vi "dfd_Multirate Filter Param Estimation.vi"(5 "method":u16(ring)=2 items=["Kaiser Window", "Dolph-Chebyshev Window", "Equi-Ripple", "Positive Equi-Ripple"], 7 "multirate factor":i32=4, 8 "error in (no error)":errorcluster, 9 "option":enum16{"Normal", "Nyquist", "Alias free"}(ring), 10 "roll off":dbl format="%.2f", 11 "order":i32) -> (0 "error out":errorcluster, 1 "window param":cluster{"low cutoff freq: fl":dbl, "param":dbl} {"param" format="%.2f"}, 2 "band parameters":T1[](array[typedef]), 3 "new order":i32)   [LabVIEW 2017, in "NI_DigFilter_Process.lvlib"]
uses:
  <vilib>/addons/Digital Filter Design/NI_DigFilter_Process.lvlib
  <vilib>/addons/Digital Filter Design/_Objects.llb/DFD Adv Band Spec.ctl
  <vilib>/addons/Digital Filter Design/NI_DigFilterLicensed.lvlib
panel:
  in  "band 2":T1
  # "freq"
  # "amplitude"
  # "weight"
  # "freq"
  # "amplitude"
  # "weight"
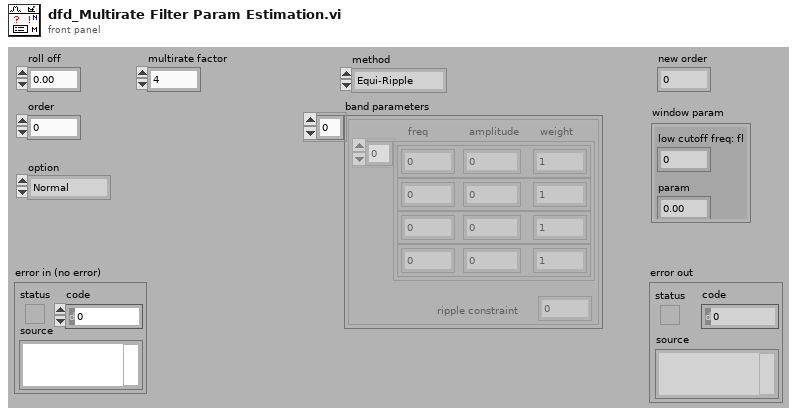
[diagram p1: front panel]
types:
  T1 = typedef "NI_DigFilterLicensed.lvlib/DFD Adv Band Spec.ctl" = cluster{"band specification":cluster{"freq":dbl, "amplitude":dbl, "weight":dbl}[], "ripple constraint":dbl}
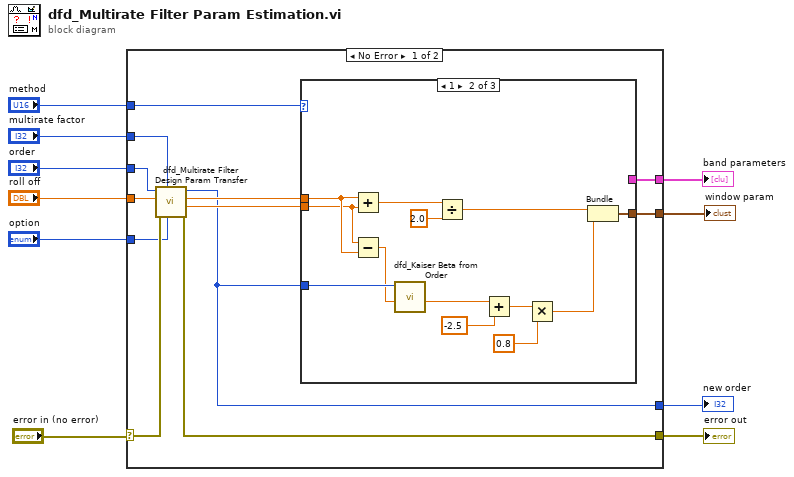
[diagram p0: block diagram]
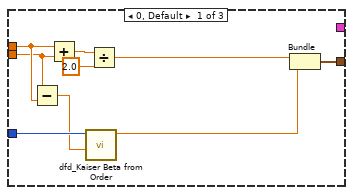
[diagram p2: hidden frame]
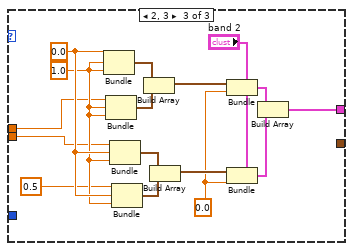
[diagram p3: hidden frame]
diagram:
  n1 = case shown="No Error" "error in (no error)" {
    selector: "error in (no error)" -> [w13 w61]
    tunnel: "roll off" -> [w18 _]
    tunnel: [w12 w61] -> w9
    tunnel: "method" -> [w22 _]
    tunnel: [w21 _] -> w7
    tunnel: "multirate factor" -> [w19 _]
    tunnel: "order" -> [w15 _]
    tunnel: [w20 _] -> w1
    tunnel: [w14 _] -> w3
    tunnel: "option" -> [w11 _]
    frame No Error {
      n2 = call <vilib>:"dfd_Multirate Filter Design Param Transfer.vi"("option"=w11, "multirate factor"=w19, "error in (no error)"=w13, "roll off"=w18, "order"=w15) -> ("error out"=w12:errorcluster, "fstop"=w17:dbl, "fpass"=w16:dbl, "new order"=w14:i32)  [unwired: 2 in, 1 out]
      n3 = case shown="1" w22 {
        tunnel: [_ _ w47] -> w21
        tunnel: w16 -> [w27 w40 w49]
        tunnel: w17 -> [w26 w39 w48]
        tunnel: w14 -> [w31 w44 _]
        tunnel: [w24 w37 _] -> w20
        frame 0, Default {
          n4 = Subtract(x=w26, y=w27) -> (x-y=w28:dbl)
          n5 = Add(x=w27, y=w26) -> (x+y=w29:dbl)
          n6 = call <vilib>:"dfd_Kaiser Beta from Order.vi"("delta f [Hz]"=w28, "order"=w31) -> ("beta"=w23:dbl)  [unwired: 9 out]
          n7 = Divide(x=w29, y=2.0) -> (x/y=w25:dbl)
          n8 = Bundle(w25, "beta"=w23) -> (w24:cluster{dbl, "beta":dbl})  [unwired: 1 out]
        }
        frame 1 {
          n9 = Add(x=w40, y=w39) -> (x+y=w42:dbl)
          n10 = Subtract(x=w39, y=w40) -> (x-y=w41:dbl)
          n11 = call <vilib>:"dfd_Kaiser Beta from Order.vi"("delta f [Hz]"=w41, "order"=w44) -> ("r [dB]"=w33:dbl)  [unwired: 9 out]
          n12 = Divide(x=w42, y=2.0) -> (x/y=w38:dbl)
          n13 = Add(x=w33, y=-2.5) -> (x+y=w36:dbl)
          n14 = Multiply(x=w36, y=0.8) -> (x*y=w32:dbl)
          n15 = Bundle(w38, w32) -> (w37:cluster{dbl, dbl})  [unwired: 1 out]
        }
        frame 2, 3 {
          w50 = 0.0
          w51 = 1.0
          w53 = 0.0
          n16 = Bundle(w53, w51, w51) -> (w60:cluster{dbl, dbl, dbl})  [unwired: 1 out]
          n17 = Bundle("fpass"=w49, w51, w51) -> (w59:cluster{"fpass":dbl, dbl, dbl})  [unwired: 1 out]
          n18 = Bundle("fstop"=w48, w53, w51) -> (w55:cluster{"fstop":dbl, dbl, dbl})  [unwired: 1 out]
          n19 = Bundle(0.5, w53, w51) -> (w56:cluster{dbl, dbl, dbl})  [unwired: 1 out]
          n20 = Build Array(w60, w59) -> (w58:cluster{"fpass":dbl, dbl, dbl}[])
          n21 = Build Array(w55, w56) -> (w57:cluster{"fstop":dbl, dbl, dbl}[])
          n22 = Bundle(cluster="band 2", "band specification"=w58, "ripple constraint"=w50) -> (w52:T1)
          n23 = Bundle(cluster="band 2", "band specification"=w57, "ripple constraint"=w50) -> (w54:T1)
          n24 = Build Array(w52, w54) -> (w47:T1[])
        }
      }
    }
    frame Error {
    }
  }
  "new order" <- w3
  "error out" <- w9
  "band parameters" <- w7
  "window param" <- w1
